vi "SpreadsheetStorage.vi"() -> ()   [LabVIEW 2015]
uses:
  <vilib>/Utility/file.llb/Write Delimited Spreadsheet (DBL).vi
panel:
  in  "AM Wave Parameters":T1
  in  "Digitalizing Parameters":T2
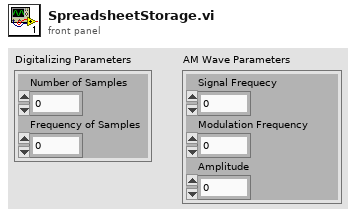
[diagram p1: front panel]
types:
  T1 = cluster{"Signal Frequecy":dbl, "Modulation Frequency":dbl, "Amplitude":dbl}
  T2 = cluster{"Number of Samples":dbl, "Frequency of Samples":dbl}
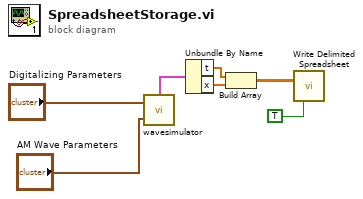
[diagram p0: block diagram]
diagram:
  n1 = call "wavesimulator.vi"("AM Wave Parameters"="AM Wave Parameters", "Digitizing Parameters"="Digitalizing Parameters") -> ("XY Graph"=w4:cluster{"t":dbl[], "x":dbl[]})  [unwired: 1 out]
  n2 = Unbundle By Name(w4) -> ("t"=w3:dbl[], "x"=w2:dbl[])
  n3 = Build Array(w3, w2) -> (w1:dbl[][])
  n4 = call-poly <vilib>:"Write Delimited Spreadsheet.vi"("2D data"=w1, "transpose? (F)"=TRUE) -> ()  [unwired: 12 in, 2 out]
